vi "BNO055 gyro recieve.vi"(9 "Write":T1, 10 "Enum":enum16{"read", "write"}(ring)) -> (1 "read":T1)   [LabVIEW 2019]
uses:
  BNO055 gyro 3axis.ctl
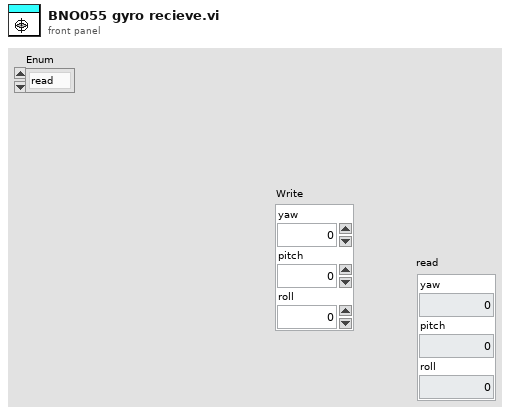
[diagram p1: front panel]
types:
  T1 = typedef "BNO055 gyro 3axis.ctl" = cluster{"yaw":dbl, "pitch":dbl, "roll":dbl}
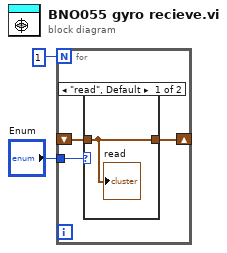
[diagram p0: block diagram]
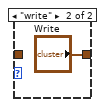
[diagram p2: hidden frame]
diagram:
  n1 = for {
    N: 1 -> [_]
    shift-right: [w4] -> _
    shift-left: _ -> [w3]
    tunnel: "Enum" -> [w5]
    n2 = case shown="\"read\", Default" w5 {
      tunnel: [w6 "Write"] -> w4
      tunnel: w3 -> [w6 _]
      frame "read", Default {
        "read" <- w6
      }
      frame "write" {
      }
    }
  }
